vi "Stop Core.vi"(10 "final error code":i32, 11 "File Actor in":refnum<class "File Actor.lvclass">) -> (3 "File Actor out":refnum<class "File Actor.lvclass">)   [LabVIEW 2014, in "File Library.lvlib" / "File Actor.lvclass"]
doc: "(<B>Filename</B>: Actor Framework.lvlib:Actor.lvclass:Stop Core.vi)\n\nDefines what the actor does before it stops. Use the <B>final error code</B> input to determine whether the actor shut down in response to an error.\n\nBy default, this method does nothing. A descendant class may override it to define behavior, such as shutting down any processes the actor initiated in its override of the Actor Core method."
uses:
  File Actor.lvclass
  reusable/Session APIs/Session Log/System Log.lvclass
  reusable/Session APIs/File Access/Config Data/Config Data.lvclass
  File Actor.lvclass/File Actor.ctl
  SuperActor/Ex Nested.lvclass/Ex Nested.ctl
  SuperActor/Read ID.vi
  SuperActor/Ex Nested.lvclass
  <userlib>/_Session Fwk/Session - Root.lvclass
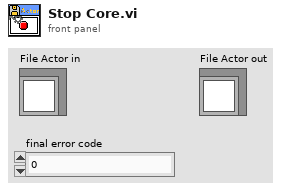
[diagram p1: front panel]
types:
  T1 = typedef "Session - Root.lvclass/Session Handle.ctl" = refnum<data-value>
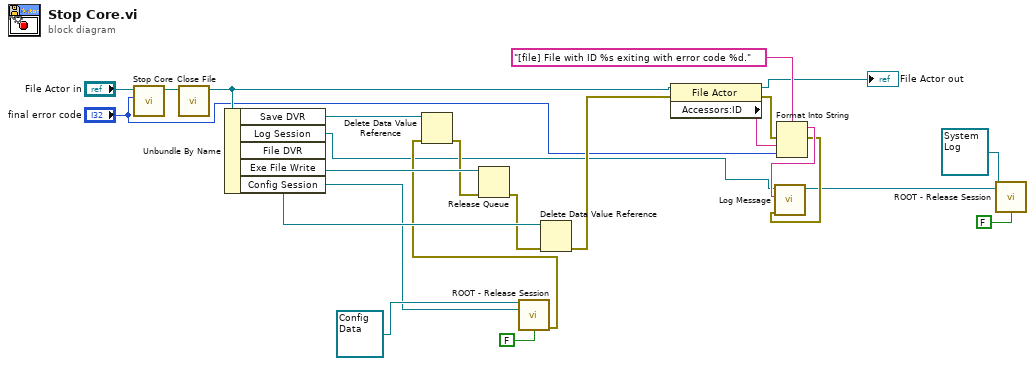
[diagram p0: block diagram]
diagram:
  n1 = call-parent "Stop Core.vi"("final error code"="final error code", "Ex Nested in"="File Actor in") -> ("Ex Nested out"=w23:refnum<class "File Actor.lvclass">)  [unwired: 9 in]
  n2 = call "Close File.vi"("File Actor in"=w23) -> ("File Actor out"=w11:refnum<class "File Actor.lvclass">)  [unwired: 9 in, 1 out]
  n3 = Unbundle By Name(w11) -> ("Save DVR"=w20:refnum<data-value>, "Log Session"=w3:T1, "File DVR"=w21:refnum<data-value>, "Exe File Write"=w19:refnum<queue>, "Config Session"=w7:T1)
  n4 = call <userlib>:"ROOT - Release Session.vi"("OBJ - Session in"=refnum<class "Config Data.lvclass"> refnum ("Config Data"), "Session Handle in"=w7, "force destroy? (F)"=FALSE) -> ("error out"=w6:errorcluster)  [unwired: 11 in, 1 out]
  n5 = Delete Data Value Reference(data value reference=w20, error in=w6) -> (error out=w15:errorcluster)  [unwired: 1 out]
  n6 = Release Queue(queue=w19, error in (no error)=w15) -> (error out=w14:errorcluster)  [unwired: 1 in, 2 out]
  n7 = Delete Data Value Reference(data value reference=w21, error in=w14) -> (error out=w13:errorcluster)  [unwired: 1 out]
  n8 = property class="File Actor"(reference=w11, error in=w13) -> (reference out=→"File Actor out":refnum<class "File Actor.lvclass">, error out=w12:errorcluster, "Accessors:ID"=w17:string)
  n9 = Format Into String(format string="[file] File with ID %s exiting with error code %d.", error in=w12, w17, "final error code") -> (resulting string=w16:string, error out=w4:errorcluster)  [unwired: 1 in]
  n10 = call "Log Message.vi"("error in"=w4, "MSG In"=w16, "session in"=w3) -> ("session out"=w1:T1)  [unwired: 7 in, 1 out]
  n11 = call <userlib>:"ROOT - Release Session.vi"("OBJ - Session in"=refnum<class "System Log.lvclass"> refnum ("Sys Log"), "Session Handle in"=w1, "force destroy? (F)"=FALSE) -> ()  [unwired: 11 in, 2 out]
